vi "svc_Fit Quadratic to Max Three Points in Array.vi"(11 "input array":dbl[](array[numeric])) -> (2 "fractional index":dbl, 3 "y extreme":dbl)   [LabVIEW 2017]
uses:
  <vilib>/Analysis/Matrix/Datatypes/RealMatrix.ctl
  <vilib>/Analysis/baseanly.llb/A x Vector.vi
  <vilib>/Analysis/baseanly.llb/Real Dot Product.vi
  <vilib>/Analysis/NI_AALBase.lvlib
  <vilib>/Analysis/Matrix/NI_Matrix.lvlib
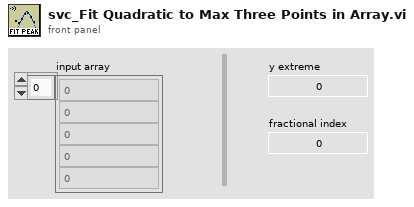
[diagram p1: front panel]
types:
  T1 = typedef "NI_Matrix.lvlib/RealMatrix.ctl" = dbl[][]
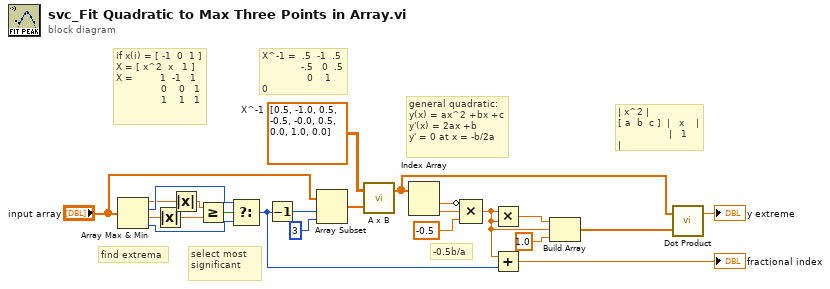
[diagram p0: block diagram]
diagram:
  w11 = T1 [[0.5, -1.0, 0.5], [-0.5, -0.0, 0.5], [0.0, 1.0, 0.0]]  # X^-1
  # "select most significant"
  # "find extrema"
  # "| x^2 |\n[ a  b  c ]  |   x    |\n                 |   1    |"
  # "X^-1 =  .5  -1  .5\n             -.5   0  .5\n               0    1   0"
  # "if x(i) = [ -1  0  1 ]\nX = [ x^2  x   1 ]\nX =         1  -1   1\n               0    0   1\n               1    1   1"
  # "general quadratic:\ny(x) = ax^2 +bx +c\ny'(x) = 2ax +b\ny' = 0 at x = -b/2a"
  # "-0.5b/a"
  n1 = Array Max & Min(array="input array") -> (max value=w4:dbl, max index (indices)=w19:i32, min value=w5:dbl, min index (indices)=w21:i32)
  n2 = Absolute Value(x=w5) -> (abs(x)=w3:dbl)
  n3 = Absolute Value(x=w4) -> (abs(x)=w2:dbl)
  n4 = Greater Or Equal?(x=w2, y=w3) -> (x >= y?=w20:bool)
  n5 = Select(t=w19, s=w20, f=w21) -> (s? t:f=w1:i32)
  n6 = Decrement(x=w1) -> (x-1=w7:i32)
  n7 = Array Subset(array="input array", index=w7, length=3) -> (w8:dbl[])
  n8 = call-poly <vilib>:"A x B.vi"("Vector"=w8, "A"=w11) -> ("A x Vector"=w15:dbl[])  [unwired: 1 out]
  n9 = Index Array(array=w15) -> (element #1=w9:dbl, element #2=w10:dbl)  [unwired: 2 in]
  n10 = Compound Arithmetic op=MULTIPLY(invert w9, w10, -0.5 ("value")) -> (w18:dbl)
  n11 = Multiply(x=w18, y=w18) -> (x*y=w13:dbl)
  n12 = Add(x=w18, y=w1) -> (x+y=→"fractional index":dbl)
  n13 = Build Array(w13, w18, 1.0 ("upper limit")) -> (w14:dbl[])
  n14 = call-poly <vilib>:"Dot Product.vi"("Y Vector"=w14, "X Vector"=w15) -> ("X * Y"=→"y extreme":dbl)  [unwired: 1 out]
